vi "Get_Tree_Item_Proj_Build.vi"(8 "error in (no error)":errorcluster, 11 "IB_Tree_Item_Proj_Build in":refnum<class "IB_Tree_Item_Proj_Build.lvclass">) -> (0 "error out":errorcluster, 2 "Dependencies":T1[](array[typedef]), 3 "IB_Tree_Item_Proj_Build out":refnum<class "IB_Tree_Item_Proj_Build.lvclass">)   [LabVIEW 2020, in "IB_Tree_Item_Proj_Build.lvclass"]
uses:
  <vilib>/AppBuilder/IB_Classes/Tree_Item_Proj_Build/IB_Tree_Item_Proj_Build.lvclass
  <vilib>/AppBuilder/IB_Classes/Tree_Item_Proj_Build/IB_Tree_Item_Proj_Build.lvclass/IB_Tree_Item_Proj_Build.ctl
  <vilib>/Utility/lvfile.llb/LVFileType.ctl
  <vilib>/Utility/lvfile.llb/NI_FileType.lvlib
  <vilib>/AppBuilder/AB_Dependency.ctl
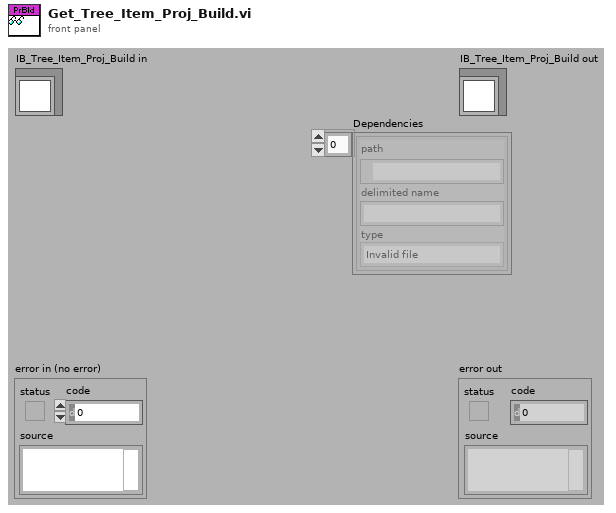
[diagram p1: front panel]
types:
  T1 = typedef "AB_Dependency.ctl" = cluster{"path":path, "delimited name":string, "type":T2}
  T2 = typedef "NI_FileType.lvlib/LVFileType.ctl" = enum32{"Invalid file", "Unknown type", "Instrument", "Control", "Polymorphic VI", "Project", "Library", "LVClass", "XControl", "XNode", "Shared library", ".NET assembly", "ActiveX interface", "CIN", "Run-time menu", "Palette menu", "Help file", "LLB", "XNode Edit Dependency", "Class Private Data Control", "Statechart", "MathScript .m file", "Ladder Diagram", "LVLibp", "XNode Build Dependency"}
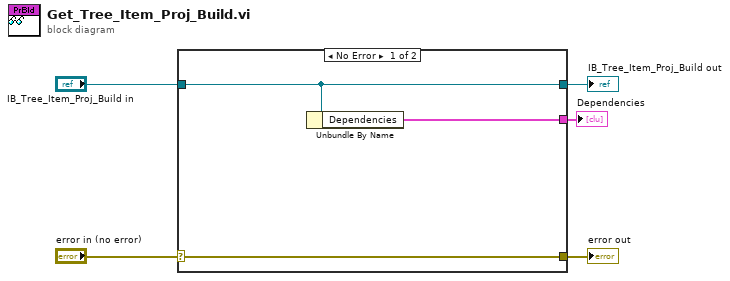
[diagram p0: block diagram]
diagram:
  n1 = case shown="No Error" "error in (no error)" {
    selector: "error in (no error)" -> [w8 w9]
    tunnel: [w8 w9] -> w4
    tunnel: [w7 w10] -> w2
    tunnel: "IB_Tree_Item_Proj_Build in" -> [w7 w10]
    tunnel: [w6 _] -> w1
    frame No Error {
      n2 = Unbundle By Name(w7) -> ("Dependencies"=w6:T1[])
    }
    frame Error {
    }
  }
  "error out" <- w4
  "IB_Tree_Item_Proj_Build out" <- w2
  "Dependencies" <- w1
